vi "Periodic Tasks.vi"(8 "error in":errorcluster) -> ()   [LabVIEW 2015]
doc: "This VI runs in parallel to other tasks. It can contain as many user-defined periodic loops as you need. These can carry out PID or other sorts of timed response."
uses:
  Common Code/Goal Vision Packet.ctl
  Common Code/Utilities/TimeManager.vi
  Common Code/Change Detect.vi
  Common Code/Change Detect Boolean.vi
  Robot Global Data.vi
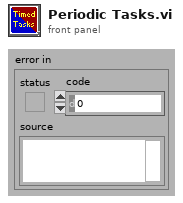
[diagram p1: front panel]
types:
  T1 = typedef "Goal Vision Packet.ctl" = cluster{"Distance":dbl, "Center X":dbl, "Center Y":dbl, "Found Target?":bool, "Robot Center":dbl, "Angle":dbl}
  T2 = typedef "Dashboard Control Data.ctl" = cluster{"Encoder Control":T3, "Steer PID output":cluster{"output high":dbl, "output low":dbl}, " Steer PID gains":cluster{"proportional gain (Kc)":dbl, "integral time (Ti, min)":dbl, "derivative time (Td, min)":dbl}, "Drivetrain Settings":T4, "Vision Packet":T1, "Dashboard Drivetrain Command":T5, "Info/Command Cluster":T7, "Ball Vision Packet":T8, "Intake Presets":T10, "Intake Encoder Control":T12, "Goal Output Range":cluster{"output high":dbl, "output low":dbl}, "Enabled Systems":T13, "Auton Presets":T14, "Pressure M":dbl, "Pressure B":dbl, "Vision Timeout":dbl, "Auto-Shift":T15, "Catapult Setpoints":T16, "Climb Presets":T17}
  T3 = typedef "Encoder Control.ctl" = cluster{"Right Tick Constant":dbl, "Left Tick Constant":dbl, "Reset?":bool, "Y Dist":cluster{"PID gains":cluster{"proportional gain (Kc)":dbl, "integral time (Ti, min)":dbl, "derivative time (Td, min)":dbl}}, "Y Stop Thresh":dbl, "Y Stop Speed":dbl}
  T4 = typedef "Drivetrain Settings.ctl" = cluster{"Gyro Tolerance":dbl, "Throttle Ramp (ms)":dbl, "Kv":dbl, "Ka":dbl, "Feed Forward P":dbl, "Feed Forward D":dbl, "Goal Vision PID gains":cluster{"proportional gain (Kc)":dbl, "integral time (Ti, min)":dbl, "derivative time (Td, min)":dbl}, "Goal Detection Window":dbl, "Creep Rate":dbl, "Vision Throttle Threshold":dbl, "Min Turn Output":dbl, "Left Batter Angle":dbl, "Right Batter Angle":dbl}
  T5 = typedef "Dashboard Drivetrain Command.ctl" = cluster{"Drivetrain Vision":T6}
  T6 = typedef "Drivetrain Vision.ctl" = cluster{"Goal Window":dbl, "Ball Window":dbl}
  T7 = typedef "Ball Tracking Command Cluster.ctl" = cluster{"Distance to Ball":dbl, "Desired Angle":dbl, "Command":enum16{"Turn to Ball", "Turn to Angle", "Get Distance"}, "Pixels from Center":dbl}
  T8 = typedef "Ball Vision Packet.ctl" = cluster{"Ball Detected?":bool, "Distance to Ball":dbl, "Desired Angle":dbl, "Pixels from Center":dbl, "Tracking mode":T9}
  T9 = typedef "Tracking Mode.ctl" = enum16{"Turn to Ball", "Turn to Angle"}
  T10 = typedef "Intake Presets.ctl" = cluster{"Intake Speed":dbl, "Outake Speed":dbl, "Angle Speed":dbl, "Angle Tolerance":dbl, "Encoder Scale":dbl, "Load Height":dbl, "Output Range":T11, "MaxCurrent":dbl, "Idle Height":dbl, "Max Height":dbl, "Reset Encoders?":bool, "PID gains":cluster{"proportional gain (Kc)":dbl, "integral time (Ti, min)":dbl, "derivative time (Td, min)":dbl}, "Drop Low Height ":dbl, "Rotation Power Max/Min":dbl, "Reset Delay":dbl, "Current Trip Delay":dbl}
  T11 = typedef "Drivetrain Output Range.ctl" = cluster{"output high":dbl, "output low":dbl}
  T12 = typedef "IntakeEcoderControl.ctl" = cluster{"Arm Tick Constant":dbl, "Reset?":bool, "Y Dist":cluster{"PID gains":cluster{"proportional gain (Kc)":dbl, "integral time (Ti, min)":dbl, "derivative time (Td, min)":dbl}}, "Y Stop Thresh":dbl, "Y Stop Speed":dbl}
  T13 = typedef "Enabled Systems.ctl" = cluster{"Shoot":bool, "Intake":bool, "DT":bool, "Gyro":bool, "100ms":bool, "US":bool}
  T14 = typedef "Autonomous Presets.ctl" = cluster{"Pitch Limit":dbl, "Roll Limit":dbl, "Start Position":dbl, "Cross Position":dbl}
  T15 = typedef "Auto Shift Cluster.ctl" = cluster{"Delay":dbl, "Speed Thresh":dbl, "Upshift Accel":dbl, "Upshift Throttle":dbl, "Upshift Throttle Accel":dbl, "Downshift Throttle":dbl, "Downshift Throttle Accel":dbl, "Pressure Threshold":dbl}
  T16 = typedef "Catapult Presets.ctl" = cluster{"Intake Danger Height":dbl, "Ball Security Delay ":dbl, "High PSI Minimum":dbl, "Shot Finish Delay":dbl, "Low PSI Minimum":dbl, "Idle Ball Security Wait ":dbl}
  T17 = typedef "Climb Presets.ctl" = cluster{"Winch Speed":dbl, "Wait until Fire":dbl, "Wait until Winch":dbl, "Wait until Stop":dbl}
  T18 = typedef "WPI_CameraDevRef.ctl" = cluster{"Camera Address":string, "CameraStatus":errorcluster}
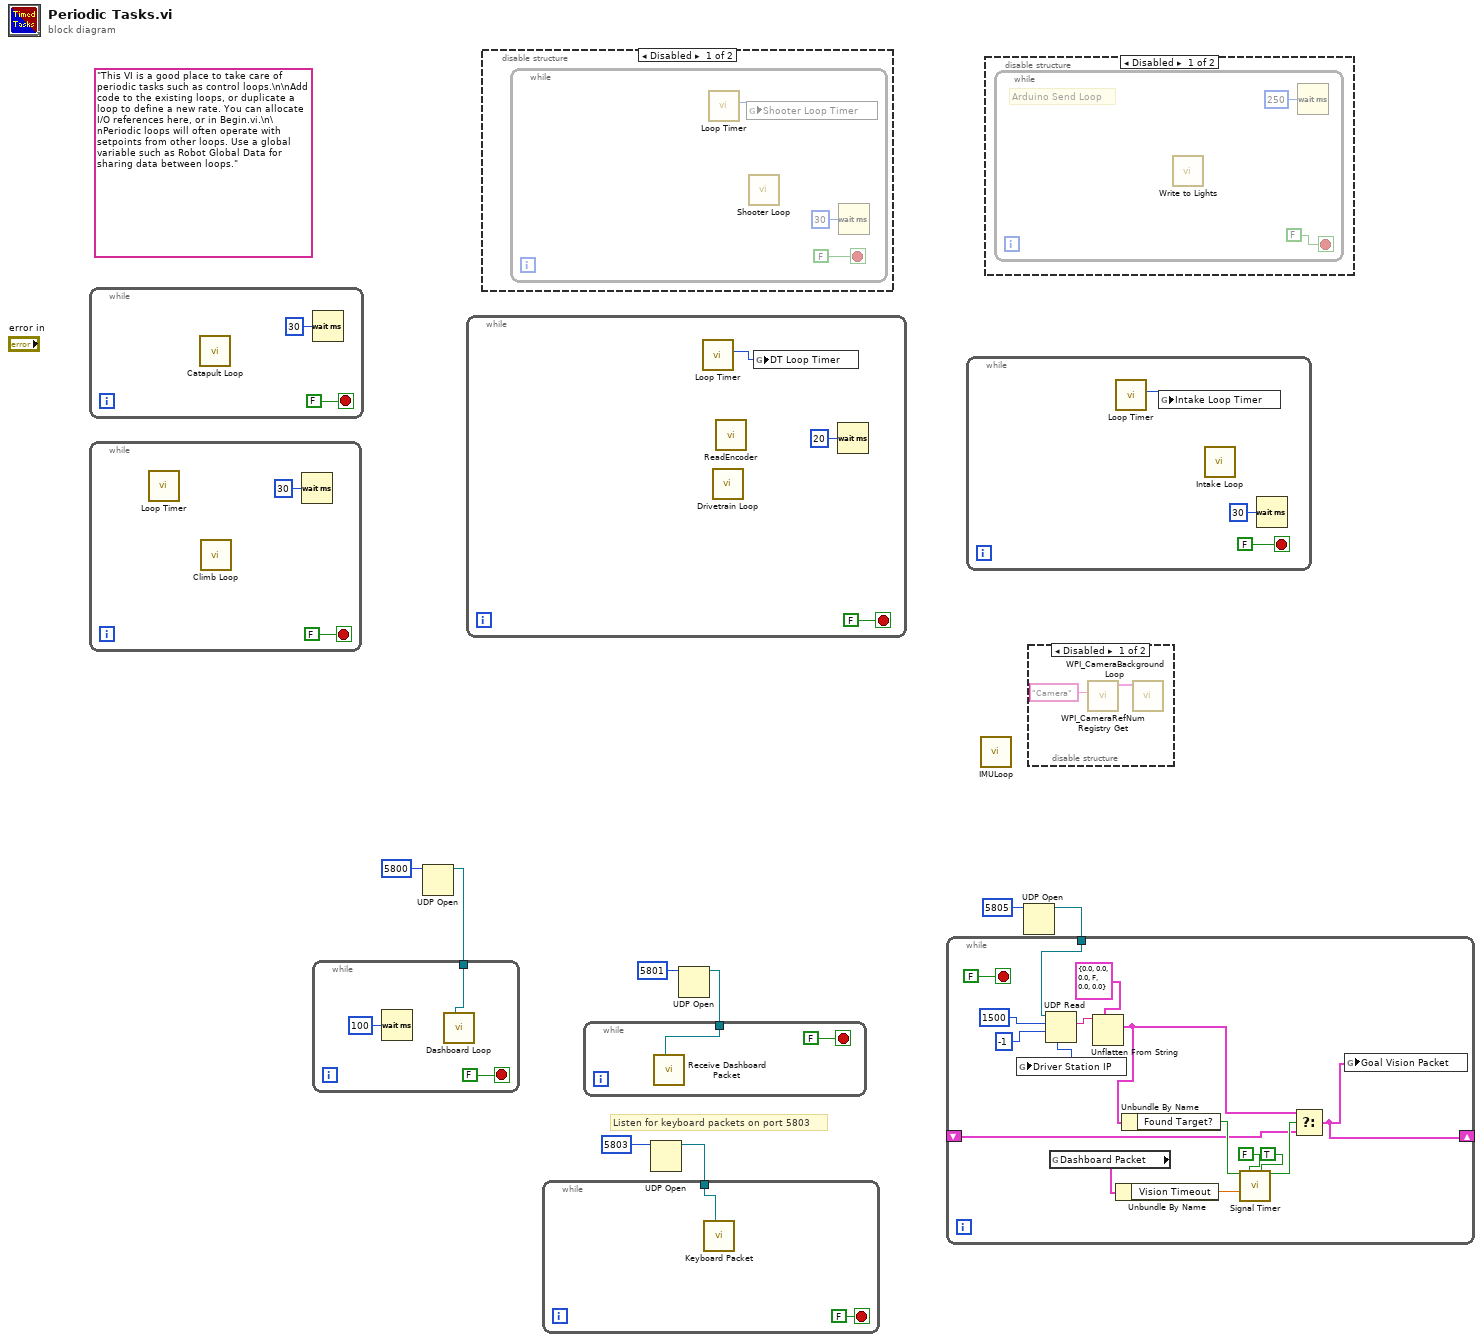
[diagram p0: block diagram]
diagram:
  (unwired) "This VI is a good place to take care of periodic tasks such as control loops.\n\nAdd code to the existing loops, or duplicate a loop to define a new rate. You can allocate I/O references here, or in Begin.vi.\n\nPeriodic loops will often operate with setpoints from other loops. Use a global variable such as Robot Global Data for sharing data between loops."
  # "Listen for keyboard packets on port 5803"
  n1 = while {
    stop <- FALSE stop-if-true
    n2 = call "Catapult Loop.vi"() -> ()  [unwired: 12 in]
    n3 = Wait (ms)(milliseconds to wait=u32 30) -> ()  [unwired: 1 out]
  }
  n4 = while {
    stop <- FALSE stop-if-true
    n5 = call "Loop Timer.vi"() -> ()  [unwired: 11 in, 1 out]
    n6 = call "Climb Loop.vi"() -> ()  [unwired: 12 in]
    n7 = Wait (ms)(milliseconds to wait=u32 30) -> ()  [unwired: 1 out]
  }
  n8 = UDP Open(11:u16 5800 ("port")) -> (port=w1:refnum<k16>)  [unwired: 4 in, 2 out]
  n9 = while {
    tunnel: w1 -> [w15]
    stop <- FALSE stop-if-true
    n10 = Wait (ms)(milliseconds to wait=u32 100) -> ()  [unwired: 1 out]
    n11 = call "Dashboard Loop.VI"("connection ID"=w15) -> ()  [unwired: 11 in]
  }
  n12 = while {
    stop <- FALSE stop-if-true
    n13 = call "Loop Timer.vi"() -> ("dt"=w16:u32)  [unwired: 11 in]
    n14 = call "Drivetrain Loop.vi"() -> ()  [unwired: 12 in]
    n15 = call "ReadEncoder.vi"() -> ()  [unwired: 11 in, 1 out]
    n16 = global write "Robot Global Data.vi" "DT Loop Timer"(w16) -> ()
    n17 = Wait (ms)(milliseconds to wait=u32 20) -> ()  [unwired: 1 out]
  }
  n18 = disable-structure shown="Disabled" {
    frame Disabled {
      n19 = while {
        stop <- FALSE stop-if-true
        n20 = call "Loop Timer.vi"() -> ("dt"=w19:u32)  [unwired: 11 in]
        n21 = global write "Robot Global Data.vi" "Shooter Loop Timer"(w19) -> ()
        n22 = call "Shooter Loop.vi"() -> ()  [unwired: 12 in]
        n23 = Wait (ms)(milliseconds to wait=u32 30) -> ()  [unwired: 1 out]
      }
    }
    frame Enabled {
    }
  }
  n24 = UDP Open(11:u16 5803 ("port")) -> (port=w5:refnum<k16>)  [unwired: 4 in, 2 out]
  n25 = while {
    tunnel: w5 -> [w22]
    stop <- FALSE stop-if-true
    n26 = call "Keyboard Packet.vi"("connection ID"=w22) -> ()  [unwired: 11 in]
  }
  n27 = UDP Open(11:u16 5801 ("port")) -> (port=w8:refnum<k16>)  [unwired: 4 in, 2 out]
  n28 = while {
    tunnel: w8 -> [w24]
    stop <- FALSE stop-if-true
    n29 = call "Receive Dashboard Packet.vi"("connection ID"=w24) -> ()  [unwired: 11 in]
  }
  n30 = while {
    stop <- FALSE stop-if-true
    n31 = call "Loop Timer.vi"() -> ("dt"=w26:u32)  [unwired: 11 in]
    n32 = global write "Robot Global Data.vi" "Intake Loop Timer"(w26) -> ()
    n33 = call "Intake Loop.vi"() -> ()  [unwired: 12 in]
    n34 = Wait (ms)(milliseconds to wait=u32 30) -> ()  [unwired: 1 out]
  }
  n35 = call "IMULoop.vi"() -> ()  [unwired: 12 in]
  n36 = disable-structure shown="Disabled" {
    frame Disabled {
      n37 = while {
        stop <- FALSE stop-if-true
        # "Arduino Send Loop"
        n38 = call "Write to Lights.vi"() -> ()  [unwired: 12 in]
        n39 = Wait (ms)(milliseconds to wait=u32 250) -> ()  [unwired: 1 out]
      }
    }
    frame Enabled {
    }
  }
  n40 = UDP Open(11:u16 5805 ("port")) -> (port=w4:refnum<k16>)  [unwired: 4 in, 2 out]
  n41 = while {
    tunnel: w4 -> [w46]
    shift-right: [w39] -> _
    shift-left: _ -> [w32]
    stop <- FALSE stop-if-true
    n42 = UDP Read(connection ID=w46, max size (548)=1500, timeout ms (25000)=-1) -> (data out=w45:string, 6:w44:u32)  [unwired: 1 in, 3 out]
    n43 = global write "Robot Global Data.vi" "Driver Station IP"(w44) -> ()
    n44 = global read "Robot Global Data.vi" "Dashboard Packet"() -> (w35:T2)
    n45 = Unflatten From String(type=T1 {"Distance"=0.0, "Center X"=0.0, "Center Y"=0.0, "Found Target?"=FALSE, "Robot Center"=0.0, "Angle"=0.0} ("Goal Vision Packet"), binary string=w45) -> (value=w41:T1)  [unwired: 3 in, 2 out]
    n46 = Unbundle By Name(w35) -> ("Vision Timeout"=w36:dbl)
    n47 = Unbundle By Name(w41) -> ("Found Target?"=w37:bool)
    n48 = call "Signal Timer.vi"("Input"=w37, "Edge"=FALSE, "Interval"=w36, "Pull"=TRUE) -> ("Filtered Output"=w38:bool)  [unwired: 11 in]
    n49 = Select(t=w41, s=w38, f=w32) -> (s? t:f=w39:T1)
    n50 = global write "Robot Global Data.vi" "Goal Vision Packet"(w39) -> ()
  }
  n51 = disable-structure shown="Disabled" {
    frame Disabled {
      n52 = call <vilib>:"WPI_CameraRefNum Registry Get.vi"("refnum name"="Camera") -> ("CameraDevRef"=w47:T18)  [unwired: 9 in, 1 out]
      n53 = call <vilib>:"WPI_CameraBackground Loop.vi"("CameraDevRef"=w47) -> ()  [unwired: 11 in]
    }
    frame Enabled {
    }
  }
